vi "NormalizeArray.vi"(1 "array":dbl[](array[numeric])) -> (0 "normalized array":dbl[](array[numeric]))   [LabVIEW 2015]
panel:
  # "Similar to WPI_RobotDriveNormalize 4.vi, this\ntakes an array of values and if any are outside\n-1 to 1, it scales them all to be within -1 to 1."
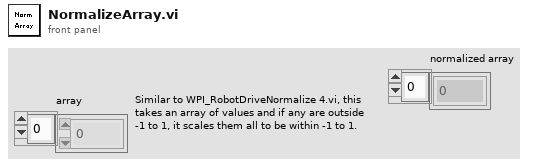
[diagram p1: front panel]
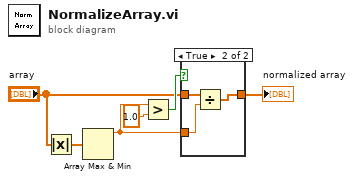
[diagram p0: block diagram]
diagram:
  n1 = Absolute Value(x="array") -> (abs(x)=w2:dbl[])
  n2 = Array Max & Min(array=w2) -> (max value=w4:dbl)  [unwired: 3 out]
  n3 = Greater?(x=w4, y=1.0) -> (0:w5:bool)
  n4 = case shown="True" w5 {
    tunnel: w4 -> [_ w10]
    tunnel: [w7 w9] -> w6
    tunnel: "array" -> [w7 w8]
    frame False {
    }
    frame True {
      n5 = Divide(x=w8, y=w10) -> (x/y=w9:dbl[])
    }
  }
  "normalized array" <- w6
